vi "FTW-CodeGen-FindGObjects.vi"(0 "GObject to Traverse":refnum<vi>, 5 "Class Name":string, 11 "error in":errorcluster) -> (6 "GObject Instances":refnum<vi>[](array[refnum]), 15 "error out":errorcluster)   [LabVIEW 2012, in "FTW-CodeGen.lvlib"]
uses:
  FTW-CodeGen.lvlib
panel:
  # "Inputs"
  # "Outputs"
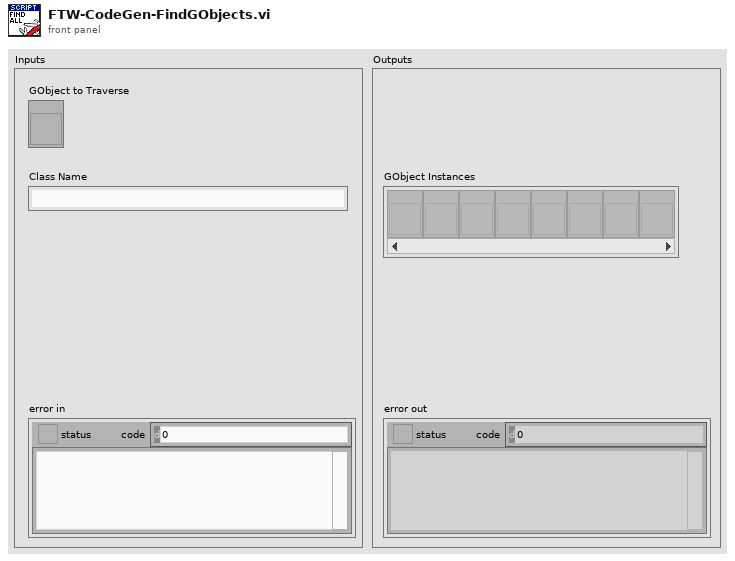
[diagram p1: front panel]
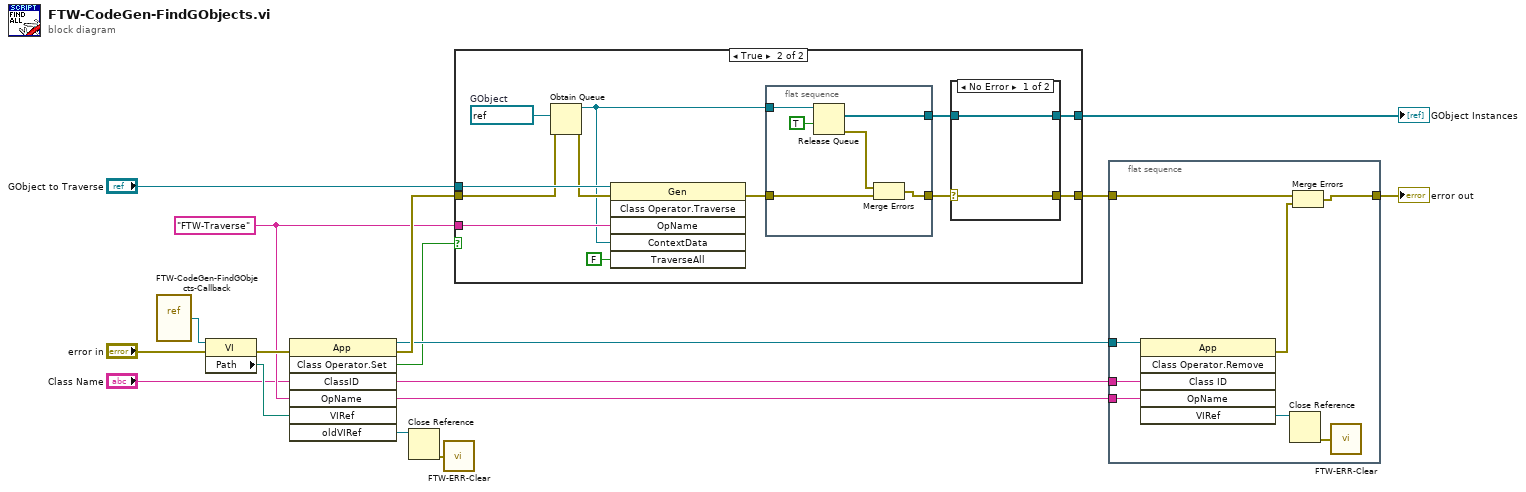
[diagram p0: block diagram]
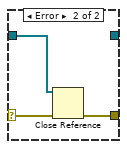
[diagram p3: hidden frame]
diagram:
  w4 = "FTW-Traverse" ("Operator Name")
  n1 = vi-ref "FTW-CodeGen-FindGObjects-Callback.vi"() -> (w11:refnum<vi>)
  n2 = property class="VI"(reference=w11, error in="error in") -> (error out=w8:errorcluster, "Path"=w10:path)  [unwired: 1 out]
  n3 = invoke class="App" method="Class Operator.Set"(error in=w8, "ClassID"="Class Name", "OpName"=w4, "VIRef"=w10) -> (reference out=w13:refnum<vi>, error out=w15:errorcluster, "SetClassOp"=w12:bool, "oldVIRef"=w2:refnum<vi>)  [unwired: 3 in, 3 out]
  n4 = Close Reference(reference=w2) -> (error out=w1:errorcluster)  [unwired: 1 in]
  n5 = call "FTW-ERR-Clear.vi"("error to snuff"=w1) -> ()  [unwired: 1 out]
  n6 = case shown="True" w12 {
    tunnel: w15 -> [w16 w25]
    tunnel: "GObject to Traverse" -> [_ w27]
    tunnel: w4 -> [_ w26]
    tunnel: [w16 w19] -> w6
    tunnel: [_ w18] -> w5
    frame False {
    }
    frame True {
      w17 = refnum<vi> refnum  # GObject
      n7 = Obtain Queue(element data type=w17, error in (no error)=w25) -> (queue out=w23:refnum<queue>, error out=w24:errorcluster)  [unwired: 3 in, 1 out]
      n8 = invoke class="Gen" method="Class Operator.Traverse"(reference=w27, error in=w24, "OpName"=w26, "ContextData"=w23, "TraverseAll"=FALSE ("Traverse All")) -> (error out=w22:errorcluster)  [unwired: 1 in, 5 out]
      n9 = flat-sequence {
        tunnel: w23 -> [w32]
        tunnel: w22 -> [w34]
        tunnel: [w29] -> w21
        tunnel: [w33] -> w20
        frame #0 {
          n10 = Release Queue(queue=w32, force destroy? (F)=TRUE) -> (remaining elements=w29:refnum<vi>[], error out=w30:errorcluster)  [unwired: 1 in, 1 out]
          n11 = Merge Errors(w30, w34) -> (w33:errorcluster)
        }
      }
      n12 = case shown="No Error" w20 {
        selector: w20 -> [w36 w39]
        tunnel: w21 -> [w35 w37]
        tunnel: [w36 w38] -> w19
        tunnel: [w35 _] -> w18
        frame No Error {
        }
        frame Error {
          n13 = Close Reference(reference=w37, error in (no error)=w39) -> (error out=w38:errorcluster)
        }
      }
    }
  }
  "GObject Instances" <- w5
  n14 = flat-sequence {
    tunnel: w13 -> [w47]
    tunnel: [w44] -> w7
    tunnel: w6 -> [w45]
    tunnel: "Class Name" -> [w43]
    tunnel: w4 -> [w42]
    frame #0 {
      n15 = invoke class="App" method="Class Operator.Remove"(reference=w47, "Class ID"=w43, "OpName"=w42) -> (error out=w41:errorcluster, "VIRef"=w46:refnum<vi>)  [unwired: 3 in, 4 out]
      n16 = Close Reference(reference=w46) -> (error out=w40:errorcluster)  [unwired: 1 in]
      n17 = Merge Errors(w45, w41) -> (w44:errorcluster)
      n18 = call "FTW-ERR-Clear.vi"("error to snuff"=w40) -> ()  [unwired: 1 out]
    }
  }
  "error out" <- w7
